vi "Read Buffers.vi"(8 "error in (no error)":errorcluster, 11 "BufferMap in":refnum<data-value>) -> (0 "error out":errorcluster, 1 "Names":string[](array[string]), 2 "Buffers":refnum<data-value>[](array[refnum]), 3 "BufferMap":refnum<data-value>)   [LabVIEW 2013, in "CircularBuffer.lvlib" / "VariantBufferMap.lvclass"]
uses:
  VariantBufferMap.lvclass
  VariantBuffer/VariantBuffer.lvclass
  VariantBufferMap.lvclass/VariantBufferMap.ctl
  VariantBuffer/WriteBufferError.vi
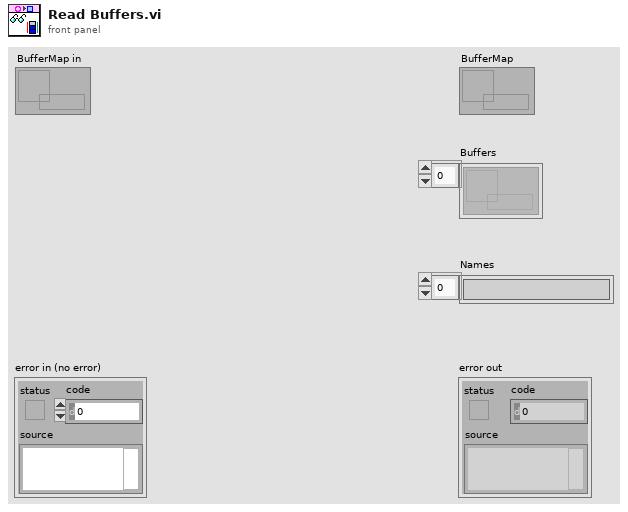
[diagram p1: front panel]
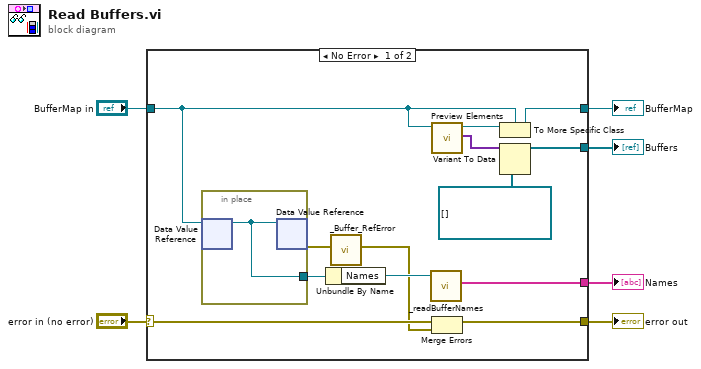
[diagram p0: block diagram]
diagram:
  n1 = case shown="No Error" "error in (no error)" {
    selector: "error in (no error)" -> [w11 w22]
    tunnel: [w10 w22] -> w5
    tunnel: [w8 w21] -> w3
    tunnel: "BufferMap in" -> [w9 w21]
    tunnel: [w16 _] -> w2
    tunnel: [w14 _] -> w1
    frame No Error {
      n2 = in-place {
        in-place-border: [w20] -> w19
        n3 = in-place-dvr #1(w9) -> (w20:refnum<class "VariantBufferMap.lvclass">)  [unwired: 1 out]
        n4 = in-place-dvr #1(w20) -> (w12:errorcluster)  [unwired: 1 out]
      }
      n5 = Unbundle By Name(w19) -> ("Names"=w17:refnum<data-value>)
      n6 = call "_Buffer_RefError.vi"("error in (no error)"=w12) -> ("error out"=w7:errorcluster)  [unwired: 10 in]
      n7 = call "_readBufferNames.vi"("Data Value Reference in"=w17) -> ("Names"=w16:string[])  [unwired: 9 in, 1 out]
      n8 = call "Preview Elements.vi"("ByteBuffer in"=w9) -> ("elements"=w15:variant[], "ByteBuffer"=w18:refnum<data-value>)  [unwired: 8 in, 1 out]
      n9 = Merge Errors(w11, w7) -> (w10:errorcluster)
      n10 = To More Specific Class(target class=w9, reference=w18) -> (specific class reference=w8:refnum<data-value>)  [unwired: 1 in, 1 out]
      n11 = Variant To Data(type=refnum<data-value>[] [] ("Buffers"), Variant=w15) -> (data=w14:refnum<data-value>[])  [unwired: 1 in, 1 out]
    }
    frame Error {
    }
  }
  "error out" <- w5
  "BufferMap" <- w3
  "Buffers" <- w1
  "Names" <- w2
